vi "Sender UI.vi"(11 "error in (no error)":errorcluster) -> (15 "error out":errorcluster)   [LabVIEW 2021, in "Sender.lvclass"]
uses:
  Sender.lvclass
  Controls/Operation.ctl
  Controls/State Cluster.ctl
  Controls/Sender Data Cluster.ctl
  Communication/Communication.lvclass
  Receiver/Receiver UI.vi
  Receiver/Receiver.lvclass
panel:
  in  "Data Type":string(combo)
  in  "Send":bool
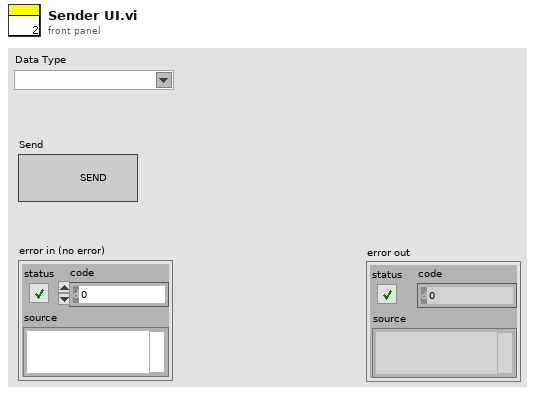
[diagram p1: front panel]
types:
  T1 = typedef "Sender Data Cluster.ctl" = cluster{"user event out":refnum<user-event>, "Selected Data Type":string}
  T2 = typedef "State Cluster.ctl" = cluster{"State":string, "Data":variant}
  T3 = typedef "Operation.ctl" = enum16{"Create", "Enqueue", "Enqueue N", "Enstack", "Dequeue", "Flush", "Release"}
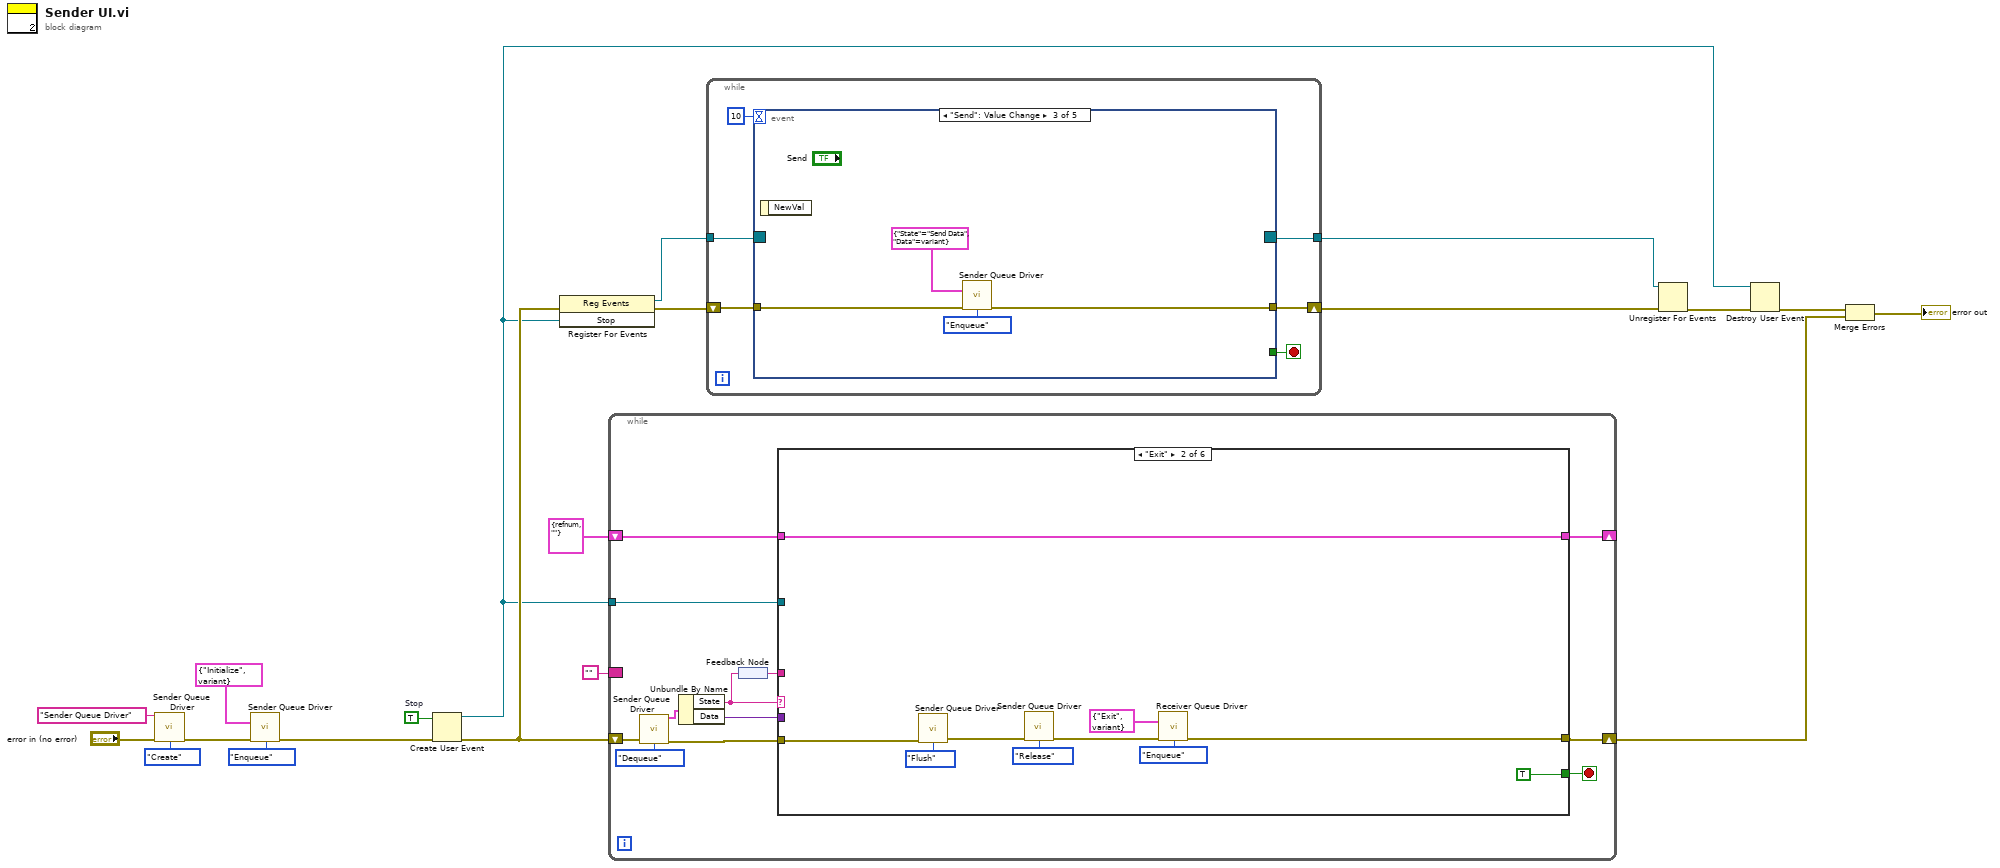
[diagram p0: block diagram]
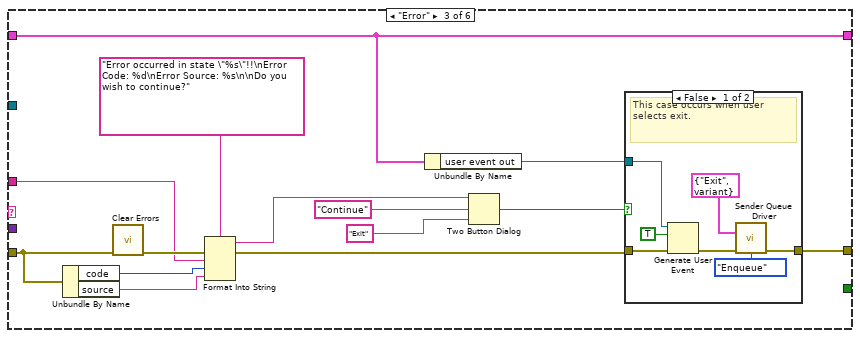
[diagram p3: hidden frame]
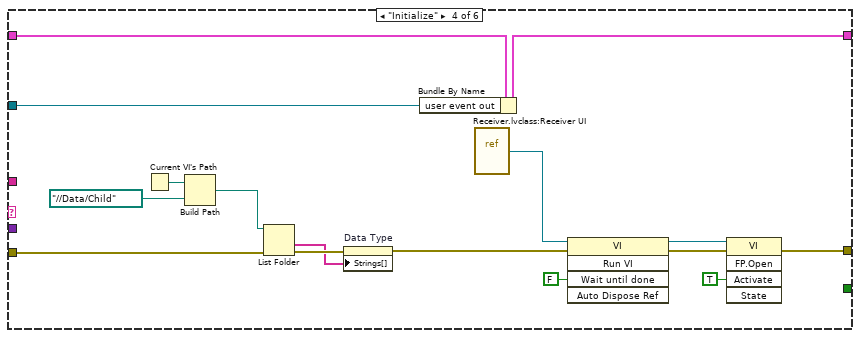
[diagram p5: hidden frame]
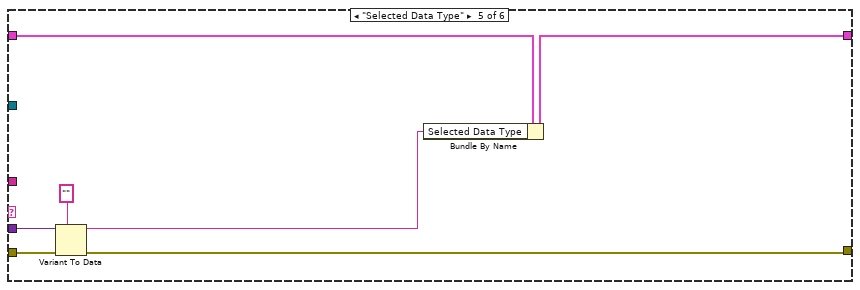
[diagram p6: hidden frame]
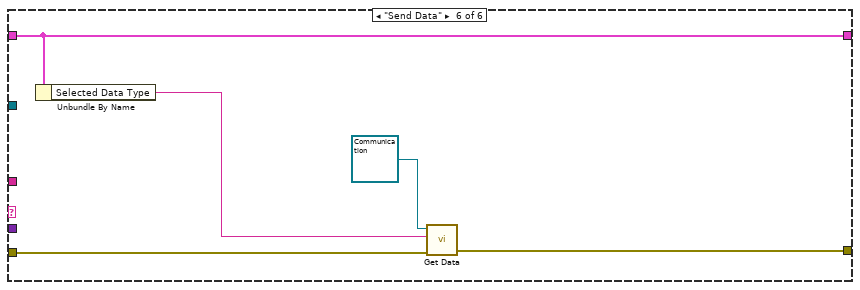
[diagram p7: hidden frame]
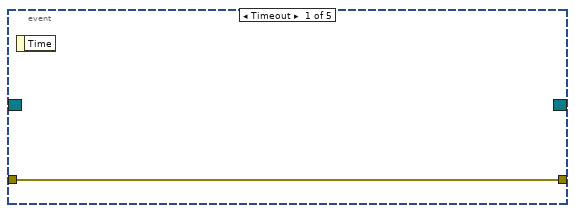
[diagram p8: hidden frame]
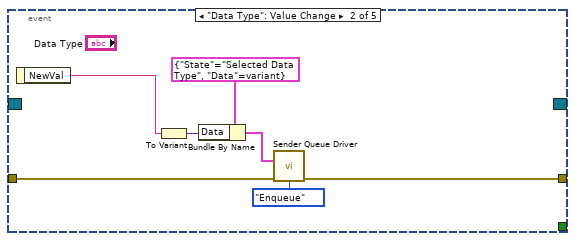
[diagram p9: hidden frame]
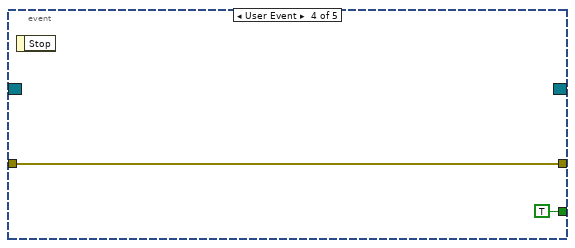
[diagram p10: hidden frame]
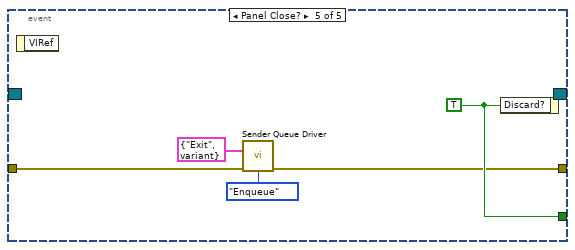
[diagram p11: hidden frame]
diagram:
  w13 = TRUE  # Stop
  n1 = call "Sender Queue Driver.vi"("Queue Name"="Sender Queue Driver", "error in (no error)"="error in (no error)", "Operations"=Operation."Create") -> ("error out"=w18:errorcluster)  [unwired: 11 in, 1 out]
  n2 = call "Sender Queue Driver.vi"("State"=T2 {"State"="Initialize", "Data"=variant}, "error in (no error)"=w18, "Operations"=Operation."Enqueue") -> ("error out"=w1:errorcluster)  [unwired: 11 in, 1 out]
  n3 = Create User Event(user event datatype=w13, error in=w1) -> (user event=w5:refnum<user-event>, error out=w12:errorcluster)
  n4 = register-events(error in=w12, w5) -> (reference out=w10:refnum<event-registration>, error out=w11:errorcluster)  [unwired: 1 in]
  n5 = while {
    shift-right: [w25] -> w3
    shift-left: w12 -> [w31]
    border: "" -> [_]
    shift-right: [w22] -> _
    shift-left: T1 {"user event out"=refnum, "Selected Data Type"=""} -> [w23]
    tunnel: w5 -> [w21]
    stop <- w24 stop-if-true
    n6 = call "Sender Queue Driver.vi"("error in (no error)"=w31, "Operations"=Operation."Dequeue") -> ("Dequeued Element"=w30:T2, "error out"=w28:errorcluster)  [unwired: 12 in]
    n7 = Unbundle By Name(w30) -> ("State"=w27:string, "Data"=w29:variant)
    n8 = feedback-in #1(w27) -> ()
    n9 = feedback #1() -> (w26:string)
    n10 = case shown="\"Exit\"" w27 {
      tunnel: w29 -> [_ _ _ _ w88 _]
      tunnel: w28 -> [w34 w43 w51 w77 w89 w94]
      tunnel: w26 -> [_ _ w47 _ _ _]
      tunnel: [w34 w37 w50 w69 w86 w93] -> w25
      tunnel: [_ TRUE _ _ _ _] -> w24
      tunnel: w23 -> [w33 w39 w46 w82 w85 w91]
      tunnel: [w33 w39 w46 w81 w84 w91] -> w22
      tunnel: w21 -> [_ _ _ w80 _ _]
      frame Default {
      }
      frame "Exit" {
        n11 = call "Sender Queue Driver.vi"("error in (no error)"=w43, "Operations"=Operation."Flush") -> ("error out"=w42:errorcluster)  [unwired: 12 in, 1 out]
        n12 = call "Sender Queue Driver.vi"("error in (no error)"=w42, "Operations"=Operation."Release") -> ("error out"=w38:errorcluster)  [unwired: 12 in, 1 out]
        n13 = call "Receiver Queue Driver.vi"("State"=T2 {"State"="Exit", "Data"=variant}, "error in (no error)"=w38, "Operations"=Operation."Enqueue") -> ("error out"=w37:errorcluster)  [unwired: 11 in, 1 out]
      }
      frame "Error" {
        n14 = Unbundle By Name(w51) -> ("code"=w49:i32, "source"=w48:string)
        n15 = call <vilib>:"Clear Errors.vi"("error in (no error)"=w51) -> ("error out"=w58:errorcluster)  [unwired: 5 in, 1 out]
        n16 = Format Into String(format string="Error occurred in state \"%s\"!!\nError Code: %d\nError Source: %s\n\nDo you wish to continue?", error in=w58, w47, w49, w48) -> (resulting string=w56:string, error out=w53:errorcluster)  [unwired: 1 in]
        n17 = Unbundle By Name(w46) -> ("user event out"=w45:refnum<user-event>)
        n18 = Two Button Dialog(message=w56, 1:"Exit" ("F button name (\"Cancel\")"), 2:"Continue" ("T button name (\"OK\")")) -> (T button?=w52:bool)
        n19 = case shown="False" w52 {
          tunnel: w53 -> [w65 w66]
          tunnel: [w62 w66] -> w50
          tunnel: w45 -> [w59 _]
          frame False {
            # "This case occurs when user selects exit."
            n20 = Generate User Event(user event=w59, event data cluster=TRUE ("event data"), error in=w65) -> (error out=w63:errorcluster)  [unwired: 1 in, 1 out]
            n21 = call "Sender Queue Driver.vi"("State"=T2 {"State"="Exit", "Data"=variant}, "error in (no error)"=w63, "Operations"=Operation."Enqueue") -> ("error out"=w62:errorcluster)  [unwired: 11 in, 1 out]
          }
          frame True {
            # "This case occurs when user selects to continue."
          }
        }
      }
      frame "Initialize" {
        n22 = Current VI's Path() -> (path=w79:path)
        n23 = Build Path(base path=w79, name or relative path=path "../../Data/Child") -> (appended path=w76:path)
        n24 = List Folder(path=w76, error in=w77) -> (folder names=w74:string[], error out=w75:errorcluster)  [unwired: 2 in, 2 out]
        n25 = property on="Data Type" class="CmbBox"(error in=w75, "Strings[]"=w74) -> (error out=w72:errorcluster)  [unwired: 1 in, 1 out]
        n26 = Bundle By Name(cluster=w82, "user event out"=w80) -> (w81:T1)
        n27 = vi-ref "Receiver.lvclass:Receiver UI.vi"() -> (w73:refnum<vi>)
        n28 = invoke class="VI" method="Run VI"(reference=w73, error in=w72, "Wait until done"=FALSE ("Wait Until Done")) -> (reference out=w68:refnum<vi>, error out=w71:errorcluster)  [unwired: 2 in, 3 out]
        n29 = invoke class="VI" method="FP.Open"(reference=w68, error in=w71, "Activate"=TRUE ("Activate?")) -> (error out=w69:errorcluster)  [unwired: 2 in, 4 out]
      }
      frame "Selected Data Type" {
        n30 = Variant To Data(error in=w89, type="", Variant=w88) -> (data=w83:string, error out=w86:errorcluster)
        n31 = Bundle By Name(cluster=w85, "Selected Data Type"=w83) -> (w84:T1)
      }
      frame "Send Data" {
        n32 = Unbundle By Name(w91) -> ("Selected Data Type"=w90:string)
        n33 = call "Get Data.vi"("error in (no error)"=w94, "Data Type"=w90, "Communication in"=refnum<class "Communication.lvclass"> refnum ("Communication.lvclass")) -> ("error out"=w93:errorcluster)  [unwired: 7 in, 1 out]
      }
    }
  }
  n34 = while {
    shift-right: [w97] -> w8
    shift-left: w11 -> [w98]
    tunnel: w10 -> [w99]
    tunnel: [w95] -> w6
    stop <- w96 stop-if-true
    n35 = event shown="[2] \"Send\": Value Change" {
      selector: w99 -> [_ _ _ _ _]
      dyn-events: [_ _ _ _ _] -> w95
      timeout: 10 -> [_ _ _ _ _]
      tunnel: w98 -> [w101 w108 w112 w114 w118]
      tunnel: [w101 w107 w111 w114 w117] -> w97
      tunnel: [_ _ _ TRUE ("Discard?") w119] -> w96
      event Timeout {
        n36 = event-data() -> ()  [unwired: 1 in, 1 out]
      }
      event "Data Type": Value Change {
        n37 = event-data() -> ("NewVal"=w103:string)  [unwired: 1 in]
        n38 = To Variant(anything=w103) -> (Variant=w104:variant)
        n39 = Bundle By Name(cluster=T2 {"State"="Selected Data Type", "Data"=variant} ("State"), "Data"=w104) -> (w102:T2)
        n40 = call "Sender Queue Driver.vi"("State"=w102, "error in (no error)"=w108, "Operations"=Operation."Enqueue") -> ("error out"=w107:errorcluster)  [unwired: 11 in, 1 out]
      }
      event "Send": Value Change {
        n41 = event-data() -> ()  [unwired: 1 in, 1 out]
        n42 = call "Sender Queue Driver.vi"("State"=T2 {"State"="Send Data", "Data"=variant}, "error in (no error)"=w112, "Operations"=Operation."Enqueue") -> ("error out"=w111:errorcluster)  [unwired: 11 in, 1 out]
      }
      event User Event {
        n43 = event-data() -> ()  [unwired: 1 in, 1 out]
      }
      event Panel Close? {
        w119 = TRUE ("Discard?")
        n44 = event-data() -> ()  [unwired: 1 in, 1 out]
        n45 = call "Sender Queue Driver.vi"("State"=T2 {"State"="Exit", "Data"=variant}, "error in (no error)"=w118, "Operations"=Operation."Enqueue") -> ("error out"=w117:errorcluster)  [unwired: 11 in, 1 out]
        n46 = event-data("Discard?"=w119) -> ()  [unwired: 1 in, 1 out]
      }
    }
  }
  n47 = Unregister For Events(event registration refnum=w6, error in=w8) -> (error out=w7:errorcluster)
  n48 = Destroy User Event(user event=w5, error in=w7) -> (error out=w4:errorcluster)
  n49 = Merge Errors(w4, w3) -> (→"error out":errorcluster)
